vi "N4_X01_check_mode.vi"(4 "Driver Name":T10, 5 "Delay befor,s":T6=2.0, 6 "Error Code":T9, 7 "InputParam":T7, 8 "error in":T8, 11 "DriverConnect in":T1={"InterfaceType"=enum."VISA", "OpenedSession"="", "InterfaceSettings"={"Interface"=enum."RS232", "EOS 4 read"=enum."LF (\\n)", "EOS 4 write"=enum."LF (\\n)", "TMO, ms"=10000, "Sett"=variant(cluster{"Baud Rate":u32, "Data Bits":u16, "Parity":u16, "Stop Bits":u16, "Flow Control":u16, "Eho":bool} {"Baud Rate"=75, "Data Bits"=0, "Parity"=0, "Stop Bits"=0, "Flow Control"=0, "Eho"=FALSE})}}) -> (0 "error out":T8, 3 "DriverConnect out":T1={"InterfaceType"=enum."VISA", "OpenedSession"="", "InterfaceSettings"={"Interface"=enum."RS232", "EOS 4 read"=enum."LF (\\n)", "EOS 4 write"=enum."LF (\\n)", "TMO, ms"=10000, "Sett"=variant(cluster{"Baud Rate":u32, "Data Bits":u16, "Parity":u16, "Stop Bits":u16, "Flow Control":u16, "Eho":bool} {"Baud Rate"=75, "Data Bits"=0, "Parity"=0, "Stop Bits"=0, "Flow Control"=0, "Eho"=FALSE})}})   [LabVIEW 2018]
uses:
  MOKO_LabViewLibrary/MokoLowLevel/MokoLowLovelControl/MLLC_DriverName.ctl
  MOKO_LabViewLibrary/MokoLowLevel/MokoLowLovelControl/MLLC_ErrorCode.ctl
  MOKO_LabViewLibrary/MokoLowLevel/MokoLowLovelControl/MLLC_Error.ctl
  MOKO_LabViewLibrary/MokoLowLevel/MokoLowLovelControl/MLLC_Command.ctl
  MOKO_LabViewLibrary/MokoLowLevel/MokoLowLovelControl/MLLC_Delay.ctl
  MOKO_LabViewLibrary/MokoLowLevel/MokoLowLovelControl/MLLC_ConnectCluster.ctl
  MOKO_LabViewLibrary/MokoLowLevel/MokoLowLovelControl/MLLC_InterfaceType.ctl
  MOKO_LabViewLibrary/MokoLowLevel/MokoLowLovelControl/MLLC_OpenedSession.ctl
  MOKO_LabViewLibrary/MokoLowLevel/MokoLowLovelControl/MLLC_InterfaceSettings.ctl
  MOKO_LabViewLibrary/MokoLowLevel/MokoLowLovelControl/MLLC_InterfaceKind.ctl
panel:
  in  "InputMode":T7
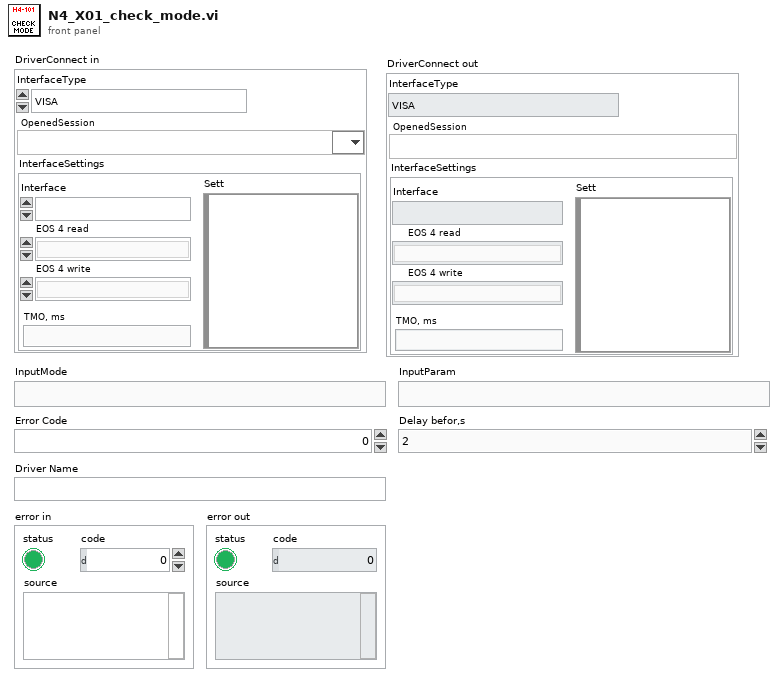
[diagram p1: front panel]
types:
  T1 = typedef "MLLC_ConnectCluster.ctl" = cluster{"InterfaceType":T2, "OpenedSession":T3, "InterfaceSettings":T4}
  T2 = typedef "MLLC_InterfaceType.ctl" = enum16{"VISA", "Prologix USB-GPIB"}
  T3 = typedef "MLLC_OpenedSession.ctl" = refnum<visa-resource-name>
  T4 = typedef "MLLC_InterfaceSettings.ctl" = cluster{"Interface":T5, "EOS 4 read":enum16{"Default (=EOS 4 write)", "CR (\\r)", "LF (\\n)", "None"}, "EOS 4 write":enum16{"CR+LF (\\r\\n)", "CR (\\r)", "LF (\\n)", "None"}, "TMO, ms":i32, "Sett":variant}
  T5 = typedef "MLLC_InterfaceKind.ctl" = enum16{"RS232", "GPIB", "USB", "Ethernet", "another"}
  T6 = typedef "MLLC_Delay.ctl" = dbl
  T7 = typedef "MLLC_Command.ctl" = string
  T8 = typedef "MLLC_Error.ctl" = errorcluster
  T9 = typedef "MLLC_ErrorCode.ctl" = u32
  T10 = typedef "MLLC_DriverName.ctl" = string
  T11 = typedef "MLLC_Response.ctl" = string
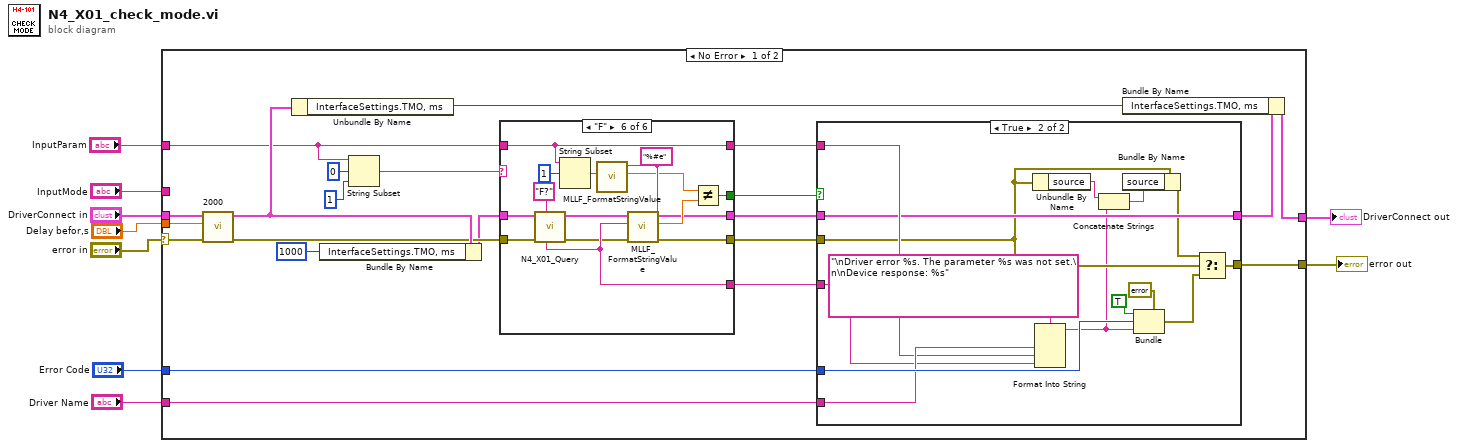
[diagram p0: block diagram]
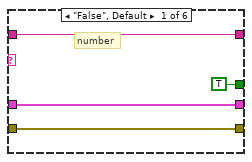
[diagram p3: hidden frame]
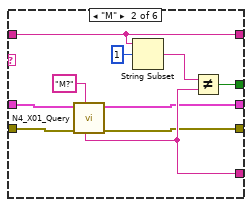
[diagram p4: hidden frame]
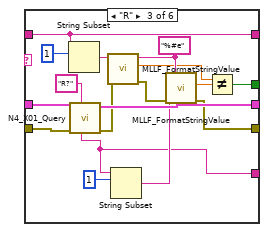
[diagram p5: hidden frame]
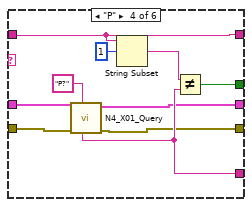
[diagram p6: hidden frame]
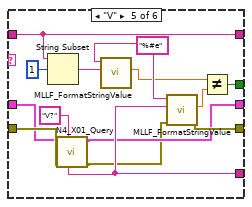
[diagram p7: hidden frame]
diagram:
  n1 = case shown="No Error" "error in" {
    selector: "error in" -> [w29 w117]
    tunnel: "DriverConnect in" -> [w30 w118]
    tunnel: "Error Code" -> [w25 _]
    tunnel: "Driver Name" -> [w24 _]
    tunnel: [w28 w118] -> w1
    tunnel: [w27 w117] -> w6
    tunnel: "InputMode" -> [_ _]
    tunnel: "InputParam" -> [w26 _]
    tunnel: "Delay befor,s" -> [w23 _]
    frame No Error {
      n2 = call "2000"("error in (no error)"=w29, "Delay Time (s)"=w23) -> ("error out"=w14:errorcluster)  [unwired: 9 in]
      n3 = Unbundle By Name(w30) -> ("InterfaceSettings.TMO, ms"=w12:i32)
      n4 = Bundle By Name(cluster=w30, "InterfaceSettings.TMO, ms"=1000 ("TMO, ms")) -> (w11:T1)
      n5 = String Subset(string=w26, offset (0)=0, length (rest)=1 ("length (rest)")) -> (substring=w18:T7)
      n6 = case shown="\"F\"" w18 {
        tunnel: w11 -> [w49 w60 w77 w87 w91 w115]
        tunnel: w14 -> [w48 w59 w76 w86 w93 w114]
        tunnel: [w49 w53 w74 w79 w90 w104] -> w21
        tunnel: [w48 w52 w68 w80 w95 w106] -> w20
        tunnel: [TRUE w57 w75 w85 w102 w113] -> w22
        tunnel: w26 -> [w50 w55 w66 w82 w96 w107]
        tunnel: [w50 w55 w66 w82 w96 w107] -> w16
        tunnel: [_ w54 w62 w81 w94 w105] -> w15
        frame "False", Default {
          # "number"
        }
        frame "M" {
          n7 = call "N4_X01_Query.vi"("Command"="M?" ("Error Query"), "error in"=w59, "DriverConnect in"=w60) -> ("error out"=w52:T8, "DriverConnect out"=w53:T1, "Response"=w54:T11)  [unwired: 6 in]
          n8 = String Subset(string=w55, offset (0)=1) -> (substring=w56:T7)  [unwired: 1 in]
          n9 = Not Equal?(x=w56, y=w54) -> (x != y?=w57:bool)
        }
        frame "R" {
          w73 = "%#e" ("format string")
          n10 = String Subset(string=w66, offset (0)=1) -> (substring=w65:T7)  [unwired: 1 in]
          n11 = call "N4_X01_Query.vi"("Command"="R?" ("Error Query"), "error in"=w76, "DriverConnect in"=w77) -> ("error out"=w70:T8, "DriverConnect out"=w74:T1, "Response"=w62:T11)  [unwired: 6 in]
          n12 = call "MLLF_FormatStringValue.vi"("error in"=w70, "String Value"=w65, "Format"=w73) -> ("error out"=w69:T8, "number"=w71:dbl)  [unwired: 6 in, 1 out]
          n13 = String Subset(string=w62, offset (0)=1) -> (substring=w63:T11)  [unwired: 1 in]
          n14 = call "MLLF_FormatStringValue.vi"("error in"=w69, "String Value"=w63, "Format"=w73) -> ("error out"=w68:T8, "number"=w72:dbl)  [unwired: 6 in, 1 out]
          n15 = Not Equal?(x=w71, y=w72) -> (x != y?=w75:bool)
        }
        frame "P" {
          n16 = call "N4_X01_Query.vi"("Command"="P?" ("Error Query"), "error in"=w86, "DriverConnect in"=w87) -> ("error out"=w80:T8, "DriverConnect out"=w79:T1, "Response"=w81:T11)  [unwired: 6 in]
          n17 = String Subset(string=w82, offset (0)=1) -> (substring=w83:T7)  [unwired: 1 in]
          n18 = Not Equal?(x=w83, y=w81) -> (x != y?=w85:bool)
        }
        frame "V" {
          w99 = "%#e" ("format string")
          n19 = String Subset(string=w96, offset (0)=1) -> (substring=w100:T7)  [unwired: 1 in]
          n20 = call "N4_X01_Query.vi"("Command"="V?" ("Error Query"), "error in"=w93, "DriverConnect in"=w91) -> ("error out"=w89:T8, "DriverConnect out"=w90:T1, "Response"=w94:T11)  [unwired: 6 in]
          n21 = call "MLLF_FormatStringValue.vi"("String Value"=w100, "Format"=w99) -> ("number"=w98:dbl)  [unwired: 7 in, 2 out]
          n22 = call "MLLF_FormatStringValue.vi"("error in"=w89, "String Value"=w94, "Format"=w99) -> ("error out"=w95:T8, "number"=w97:dbl)  [unwired: 6 in, 1 out]
          n23 = Not Equal?(x=w98, y=w97) -> (x != y?=w102:bool)
        }
        frame "F" {
          w110 = "%#e" ("format string")
          n24 = call "N4_X01_Query.vi"("Command"="F?" ("Error Query"), "error in"=w114, "DriverConnect in"=w115) -> ("error out"=w103:T8, "DriverConnect out"=w104:T1, "Response"=w105:T11)  [unwired: 6 in]
          n25 = String Subset(string=w107, offset (0)=1) -> (substring=w111:T7)  [unwired: 1 in]
          n26 = call "MLLF_FormatStringValue.vi"("String Value"=w111, "Format"=w110) -> ("number"=w109:dbl)  [unwired: 7 in, 2 out]
          n27 = call "MLLF_FormatStringValue.vi"("error in"=w103, "String Value"=w105, "Format"=w110) -> ("error out"=w106:T8, "number"=w108:dbl)  [unwired: 6 in, 1 out]
          n28 = Not Equal?(x=w109, y=w108) -> (x != y?=w113:bool)
        }
      }
      n29 = case shown="True" w22 {
        tunnel: w21 -> [w32 w41]
        tunnel: [w32 w41] -> w10
        tunnel: [w31 w33] -> w27
        tunnel: w20 -> [w31 w39]
        tunnel: w16 -> [_ w42]
        tunnel: w25 -> [_ w44]
        tunnel: w24 -> [_ w43]
        tunnel: w15 -> [_ w40]
        frame False {
        }
        frame True {
          n30 = Unbundle By Name(w39) -> ("source"=w38:string)
          n31 = Format Into String(format string="\nDriver error %s. The parameter %s was not set.\n\nDevice response: %s", w43, w42, w40) -> (resulting string=w36:string)  [unwired: 2 in, 1 out]
          n32 = Concatenate Strings(w38, w36) -> (w37:string)
          n33 = Bundle By Name(cluster=w39, "source"=w37) -> (w35:T8)
          n34 = Bundle(cluster=errorcluster {"status"=FALSE, "code"=0, "source"=""} ("error out"), "status"=TRUE ("Status"), "code"=w44, "source"=w36) -> (w34:errorcluster)
          n35 = Select(t=w35, s=w39, f=w34) -> (s? t:f=w33:T8)
        }
      }
      n36 = Bundle By Name(cluster=w10, "InterfaceSettings.TMO, ms"=w12) -> (w28:T1)
    }
    frame Error {
    }
  }
  "error out" <- w6
  "DriverConnect out" <- w1
